vi "re_LuaVIEW CIN.vi"(0 "action":T2=enum."luaversion", 1 "refnum in":refnum<vi>, 2 "supplement":string, 5 "LuaVIEW reference in":T3, 7 "index in":i32, 9 "number in":dbl format="%.2f", 11 "string in":string, 12 "boolean in":bool) -> (3 "refnum out":refnum<vi>, 4 "result":T1, 6 "LuaVIEW reference out":T3, 8 "index out":i32, 10 "number out":dbl format="%.2f", 14 "boolean out":bool, 15 "string out":string)   [LabVIEW 2013]
doc: "This VI wraps the LuaVIEW CIN. This is the only place where Lua C code is located. This VI as well as the CIN are reentrant so as to allow multiple virtual machines to execute in parallel. A small subset of actions, denoted with a leading underscore, must be called through the spinlock wrapper so as to serialize access to global state. This VI is private. It should NEVER be used directly by VIs that are not part of the LuaVIEW toolkit."
uses:
  typedefs/et_LuaVIEW CIN Actions.ctl
  typedefs/et_LuaVIEW CIN Results.ctl
  typedefs/t_LuaVIEW Reference.ctl
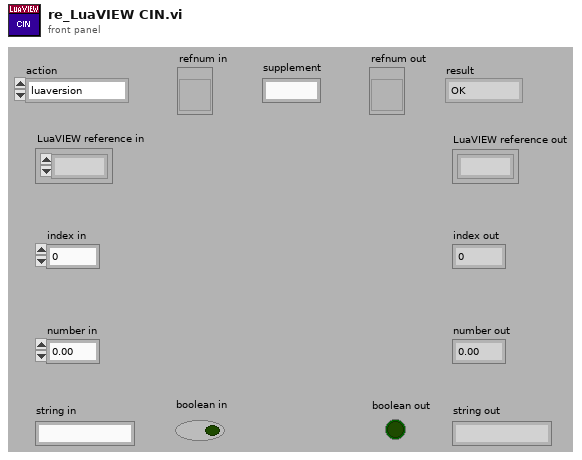
[diagram p1: front panel]
types:
  T1 = typedef "et_LuaVIEW CIN Results.ctl" = enum16{"OK", "error", "main", "call", "clonecall", "modulecall", "exportcall", "index", "yield"}
  T2 = typedef "et_LuaVIEW CIN Actions.ctl" = enum16{"checksynopsis", "_open", "_registerpublic", "_registerexport", "__never_an_error_result_ns", "luaversion", "cinversion", "_totals", "_taskcount", "pathological", "_unregnextpublic", "registryusecount", "__per_state_actions", "regsetprivate", "regsetindex", "regsetmodule", "_revokeexports", "_usepublic", "prepare", "compile", "execute", "call", "unregstaterefs", "_close", "pullboolean", "pullnumber", "pullI8", "pullU8", "pullI16", "pullU16", "pullI32", "pullU32", "pullobject", "pullrefnum", "pullstring", "pullflat", "pushflat", "pushobject", "getattribute", "setattribute", "stacktostring", "_startyieldtest", "_endyieldtest", "_pollprintbuffer", "__never_an_error_result_ps", "_pollexport", "setclone", "forcecleanup", "gettop", "clearstack", "insert", "pushboolean", "pushnumber", "pushrefnum", "pushstring", "pushnil", "pushvalue", "gettaskref", "settaskref"}
  T3 = typedef "t_LuaVIEW Reference.ctl" = refnum<k1>
  T4 = enum16{"OK", "error", "main", "call", "clonecall", "modulecall", "exportcall", "index", "yield"}
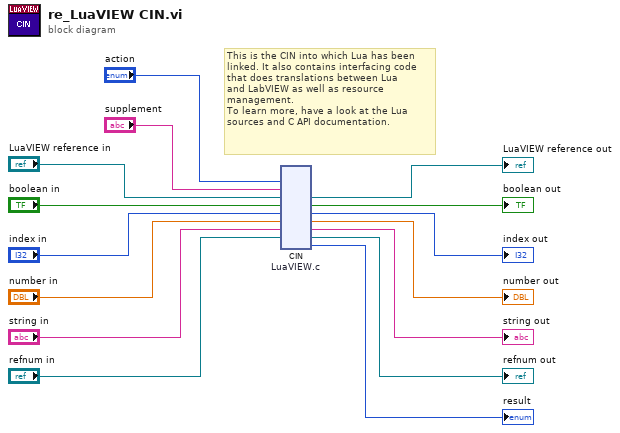
[diagram p0: block diagram]
diagram:
  # "This is the CIN into which Lua has been\nlinked. It also contains interfacing code\nthat does translations between Lua\nand LabVIEW as well as resource\nmanagement.\nTo learn more, have a look at the Lua\nsources and C API documentation."
  n1 = cin "LuaVIEW.c"("action", "supplement", "LuaVIEW reference in", "boolean in", "index in", "number in", "string in", "refnum in") -> (→"LuaVIEW reference out":refnum<k1>, →"boolean out":bool, →"index out":i32, →"number out":dbl, →"string out":string, →"refnum out":refnum<vi>, →"result":T4)  [unwired: 3 in]
